vi "Formal Check Array by Int.vi"(10 "Array Formal In":T1[](array[typedef])=[{"Variant"=[]}, {"Variant"=[1, 2, 3, 4, 5, 6, 7, 8, 9]}, {"Variant"=[]}, {"Variant"=[1, 2, 3, 4, 5, 6, 7, 8, 9]}, {"Variant"=[1, 2, 3, 4, 5, 6, 7, 8, 9]}, {"Variant"=[]}, {"Variant"=[1, 2, 3, 4, 5, 6, 7, 8, 9]}, {"Variant"=[1, 2, 3, 4, 5, 6, 7, 8, 9]}, {"Variant"=[]}], 11 "Array In":u8[](array[numeric])=[2, 0, 5, 0, 0, 9, 0, 0, 4]) -> (2 "Array Formal Out":T1[](array[typedef]), 3 "Is Modify":bool)   [LabVIEW 2015, in "Sudoku Library.lvlib"]
doc: "Created IvanLis by LabVIEW Portal\nProfile: http://labviewportal.org/memberlist.php?mode=viewprofile&u=987\neMail: IvanLisanov@gMail.com\nTelegram: https://t.me/IvanLis"
uses:
  Sudoku Library.lvlib
  TypeDef/Cell Formal.ctl
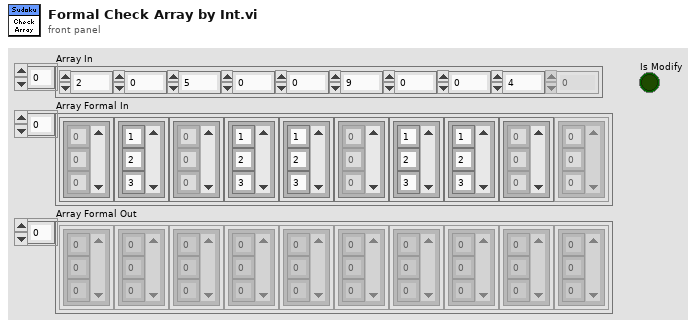
[diagram p1: front panel]
types:
  T1 = typedef "Sudoku Library.lvlib/Cell Formal.ctl" = cluster{"Variant":u8[]}
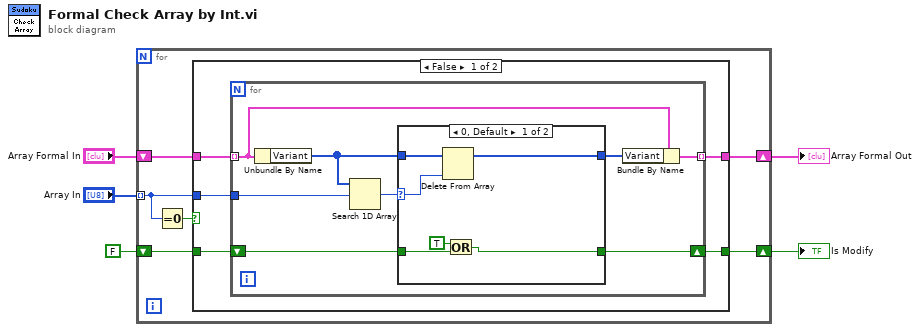
[diagram p0: block diagram]
diagram:
  n1 = for {
    shift-right: [w9] -> w3
    shift-left: "Array Formal In" -> [w10]
    tunnel: "Array In" -> [w8] mode=indexing
    shift-right: [w6] -> w1
    shift-left: FALSE -> [w7]
    n2 = Equal To 0?(x=w8) -> (x = 0?=w11:bool)
    n3 = case shown="False" w11 {
      tunnel: w10 -> [w16 w34]
      tunnel: [w14 w34] -> w9
      tunnel: w8 -> [w15 _]
      tunnel: [w12 w33] -> w6
      tunnel: w7 -> [w13 w33]
      frame False {
        n4 = for {
          tunnel: w16 -> [w21] mode=indexing
          tunnel: w15 -> [w22]
          tunnel: [w19] -> w14 mode=indexing
          shift-right: [w17] -> w12
          shift-left: w13 -> [w18]
          n5 = Unbundle By Name(w21) -> ("Variant"=w23:u8[])
          n6 = Search 1D Array(1D array=w23, element=w22) -> (index of element=w24:i32)  [unwired: 1 in]
          n7 = case shown="0, Default" w24 {
            selector: w24 -> [w29 _]
            tunnel: w23 -> [w25 w32]
            tunnel: [w30 w32] -> w20
            tunnel: w18 -> [w28 w31]
            tunnel: [w27 w31] -> w17
            frame 0, Default {
              n8 = Delete From Array(array=w25, index=w29) -> (array with subset deleted=w30:u8[])  [unwired: 1 in, 1 out]
              n9 = Or(x=TRUE, y=w28) -> (x .or. y?=w27:bool)
            }
            frame -1 {
            }
          }
          n10 = Bundle By Name(cluster=w21, "Variant"=w20) -> (w19:T1)
        }
      }
      frame True {
      }
    }
  }
  "Array Formal Out" <- w3
  "Is Modify" <- w1
